vi "Is Filled.vi"(8 "error in (no error)":errorcluster, 11 "Tool Path in":refnum<class "Tool Path.lvclass">) -> (0 "error out":errorcluster, 2 "Filled?":bool, 3 "Tool Path out":refnum<class "Tool Path.lvclass">)   [LabVIEW 2019, in "Tool Path.lvclass"]
uses:
  Tool Path.lvclass
  Tool Object/Tool Object.lvclass
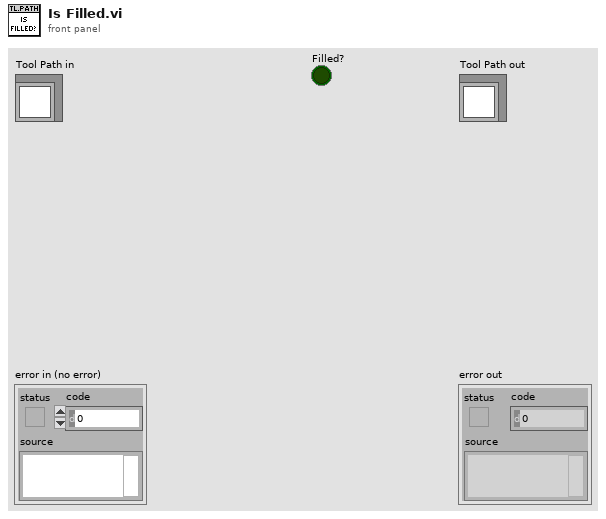
[diagram p1: front panel]
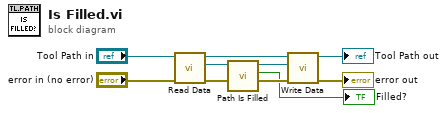
[diagram p0: block diagram]
diagram:
  n1 = call-dynamic "Read Data.vi"("error in (no error)"="error in (no error)", "Tool Path in"="Tool Path in") -> ("error out"=w2:errorcluster, "Path.lvclass"=w4:refnum<class "Path.lvclass">, "Tool Path out"=w6:refnum<class "Tool Path.lvclass">)  [unwired: 7 in]
  n2 = call "Path Is Filled.vi"("error in (no error)"=w2, "Path in"=w4) -> ("error out"=w3:errorcluster, "x != y?"=→"Filled?":bool, "Path out"=w5:refnum<class "Path.lvclass">)  [unwired: 7 in]
  n3 = call-dynamic "Write Data.vi"("error in (no error)"=w3, "Path.lvclass"=w5, "Tool Path in"=w6) -> ("error out"=→"error out":errorcluster, "Tool Path out"=→"Tool Path out":refnum<class "Tool Path.lvclass">)  [unwired: 7 in]
